vi "TableControl_1Column.vi"(0 "CtlRef":refnum<vi>, 5 "CharIn":i16, 7 "VKey":T1, 9 "ScanCode":i16) -> (6 "CharOut":i16, 15 "Discard?":bool)   [LabVIEW 2019]
uses:
  <vilib>/event_ctls.llb/eventvkey.ctl
  <vilib>/Utility/miscctls.llb/LVRowAndColumnTypeDef.ctl
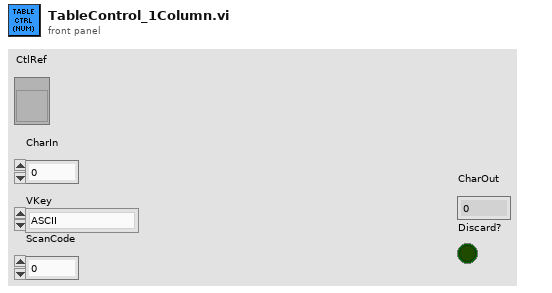
[diagram p1: front panel]
types:
  T1 = typedef "eventvkey.ctl" = enum16{"ASCII", "Enter", "Return", "Shift", "Ctrl", "Alt", "Cmd", "Opt", "Caps", "NumLock", "Clear", "Break", "Up", "Down", "Left", "Right", "Insert", "Delete", "Home", "End", "PageUp", "PageDown", "Escape", "Help", "Pause", "ScrollLock", "F1", "F2", "F3", "F4", "F5", "F6", "F7", "F8", "F9", "F10", "F11", "F12", "F13", "F14", "F15", "F16", "F17", "F18", "F19", "F20", "F21", "F22", "F23", "F24", "Play", "VolumeUp", "VolumeDown", "Mute", "Two Byte Char"}
  T2 = typedef "LVRowAndColumnTypeDef.ctl" = cluster{"Row":i32, "Column":i32}
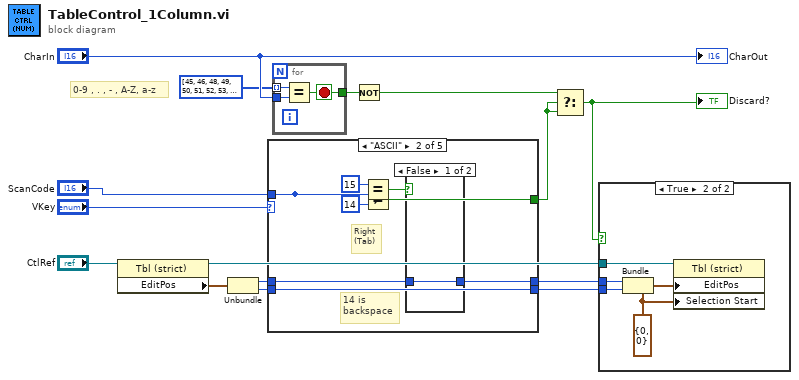
[diagram p0: block diagram]
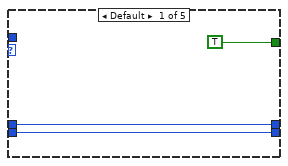
[diagram p3: hidden frame]
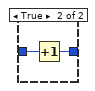
[diagram p4: hidden frame]
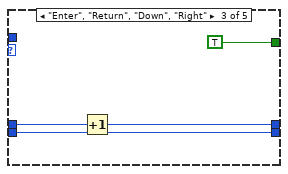
[diagram p5: hidden frame]
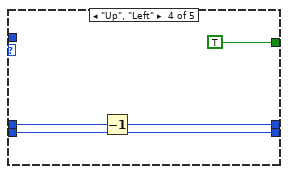
[diagram p6: hidden frame]
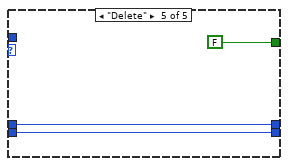
[diagram p7: hidden frame]
diagram:
  # "0-9 , . , - , A-Z, a-z"
  n1 = property on="Property Node" class="Tbl (strict)"(reference="CtlRef") -> (reference out=w12:refnum<vi>, "EditPos"=w11:T2)  [unwired: 1 in, 1 out]
  n2 = Unbundle(w11) -> ("Row"=w10:i32, "Column"=w9:i32)
  n3 = case shown="\"ASCII\"" "VKey" {
    tunnel: "ScanCode" -> [_ w24 _ _ _]
    tunnel: w10 -> [w18 w20 w33 w37 w40]
    tunnel: w9 -> [w17 w21 w31 w36 w39]
    tunnel: [w18 w19 w32 w35 w40] -> w8
    tunnel: [w17 w21 w31 w36 w39] -> w7
    tunnel: [TRUE w22 TRUE TRUE FALSE] -> w2
    frame Default {
    }
    frame "ASCII" {
      # "14 is\nbackspace"
      # "Right\n(Tab)"
      n4 = Equal?(x=i16 15, y=w24) -> (x = y?=w25:bool)
      n5 = Not Equal?(x=w24, y=i16 14 ("x")) -> (x != y?=w22:bool)
      n6 = case shown="False" w25 {
        tunnel: w20 -> [w27 w29]
        tunnel: [w27 w28] -> w19
        frame False {
        }
        frame True {
          n7 = Increment(x=w29) -> (x+1=w28:i32)
        }
      }
    }
    frame "Enter", "Return", "Down", "Right" {
      n8 = Increment(x=w33) -> (x+1=w32:i32)
    }
    frame "Up", "Left" {
      n9 = Decrement(x=w37) -> (x-1=w35:i32)
    }
    frame "Delete" {
    }
  }
  n10 = for {
    tunnel: i16[] [45, 46, 48, 49, 50, 51, 52, 53, 54, 55, 56, 57, 65, 66, 67, 68, 69, 70, 71, 72, 73, 74, 75, 76, 77, 78, 79, 80, 81, 82, 83, 84, 85, 86, 87, 88, 89, 90, 97, 98, 99, 100, 101, 102, 103, 104, 105, 106, 107, 108, 109, 110, 111, 112, 113, 114, 115, 116, 117, 118, 119, 120, 121, 122] -> [w43] mode=indexing
    tunnel: "CharIn" -> [w42]
    tunnel: [w41] -> w5
    stop <- w41 stop-if-true
    n11 = Equal?(x=w43, y=w42) -> (x = y?=w41:bool)
  }
  n12 = Not(x=w5) -> (.not. x?=w4:bool)
  n13 = Select(t=w4, s=w2, f=w2) -> (s? t:f=w3:bool)
  "Discard?" <- w3
  n14 = case shown="True" w3 {
    tunnel: w12 -> [_ w48]
    tunnel: w8 -> [_ w46]
    tunnel: w7 -> [_ w45]
    frame False {
    }
    frame True {
      w44 = T2 {"Row"=0, "Column"=0} ("Active Cell:Active Cell")
      n15 = Bundle(cluster=w44, "Row"=w46, "Column"=w45) -> (w47:T2)
      n16 = property on="Property Node" class="Tbl (strict)"(reference=w48, "EditPos"=w47, "Selection Start"=w44) -> ()  [unwired: 1 in, 2 out]
    }
  }
  "CharOut" <- "CharIn"
